vi "DSF.Engine.Memory.Cache.Transfer.Initialize Buffer.vi"(8 "error in (no error)":errorcluster, 11 "Transfer Cache in":refnum<class "DSF.Engine.Memory.Cache.Transfer.lvclass">) -> (0 "error out":errorcluster, 3 "Transfer Cache out":refnum<class "DSF.Engine.Memory.Cache.Transfer.lvclass">)   [LabVIEW 2016, in "DSF.Engine.lvlib" / "DSF.Engine.Memory.Cache.Transfer.lvclass"]
uses:
  DSF.Engine.Memory.Cache.Transfer.lvclass
  DSF.Engine.Memory.Cache.Transfer.lvclass/DSF.Engine.Memory.Cache.Transfer.ctl
  Shared/Classes/Transfer/DSF.Shared.Configuration.Transfer.lvclass/DSF.Shared.Configuration.Transfer.ctl
  Shared/Classes/Transfer/DSF.Shared.Configuration.Transfer.Get Block Descriptors.vi
  Shared/VIs/DSF.Shared.Data Type.Sizeof.1D.vi
  Shared/VIs/DSF.Shared.Data Type.Sizeof.vi
  Shared/Classes/Transfer/DSF.Shared.Configuration.Transfer.lvclass
  Buffer/DSF.Engine.Memory.Buffer.lvclass
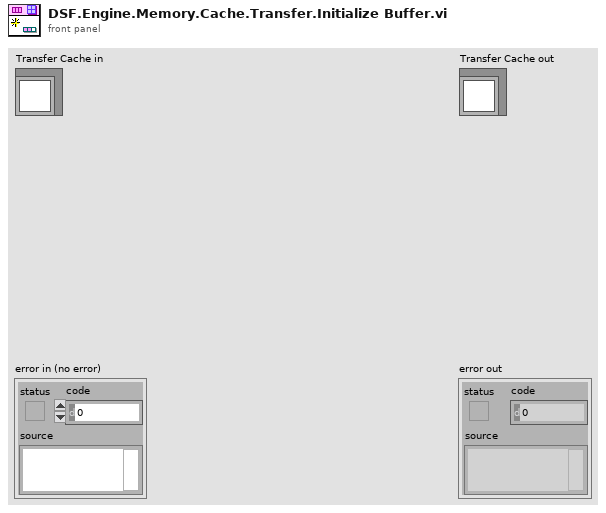
[diagram p1: front panel]
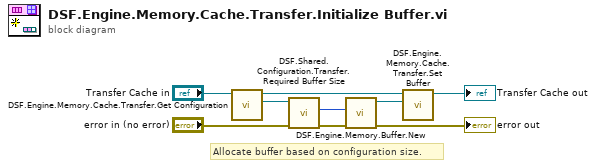
[diagram p0: block diagram]
diagram:
  # "Allocate buffer based on configuration size."
  n1 = call "DSF.Engine.Memory.Cache.Transfer.Get Configuration.vi"("Transfer Cache in"="Transfer Cache in") -> ("Transfer Configuration"=w6:refnum<class "DSF.Shared.Configuration.Transfer.lvclass">, "Transfer Cache out"=w4:refnum<class "DSF.Engine.Memory.Cache.Transfer.lvclass">)  [unwired: 9 in]
  n2 = call "DSF.Shared.Configuration.Transfer.Required Buffer Size.vi"("error in (no error)"="error in (no error)", "Transfer Configuration in"=w6) -> ("error out"=w5:errorcluster, "required buffer size"=w1:u64)  [unwired: 7 in, 1 out]
  n3 = call "DSF.Engine.Memory.Buffer.New.vi"("error in (no error)"=w5, "size"=w1) -> ("error out"=→"error out":errorcluster, "Buffer out"=w9:refnum<class "DSF.Engine.Memory.Buffer.lvclass">)  [unwired: 8 in]
  n4 = call "DSF.Engine.Memory.Cache.Transfer.Set Buffer.vi"("Buffer"=w9, "Transfer Cache in"=w4) -> ("Transfer Cache out"=→"Transfer Cache out":refnum<class "DSF.Engine.Memory.Cache.Transfer.lvclass">)  [unwired: 9 in]
